vi "registerObserver.vi"(8 "error in (no error)":errorcluster, 10 "Observer.lvclass":refnum<class "Observer.lvclass">, 11 "Subject.lvclass":refnum<class "Subject.lvclass">) -> (0 "error out":errorcluster, 3 "Subject.lvclass 2":refnum<class "Subject.lvclass">)   [LabVIEW 2020, in "Subject.lvclass"]
uses:
  Subject.lvclass
  Observer/Observer.lvclass
panel:
  # "Connector Pane"
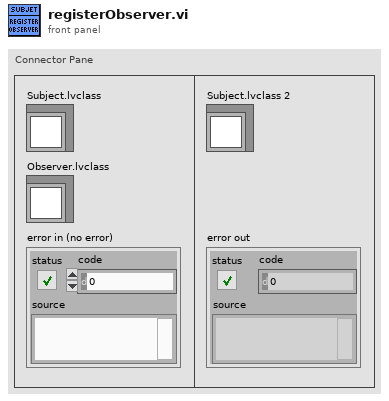
[diagram p1: front panel]
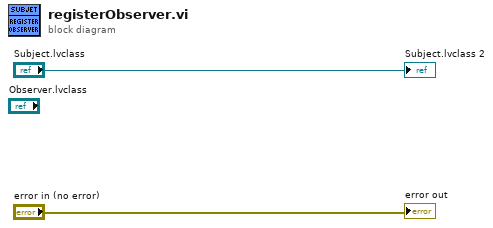
[diagram p0: block diagram]
diagram:
  "error out" <- "error in (no error)"
  "Subject.lvclass 2" <- "Subject.lvclass"
